vi "ADRextraction.vi"(8 "Path in":path) -> (10 "Error":string, 11 "Array":dbl[](array[numeric]), 12 "raw xML":string, 13 "duration":dbl[](array[numeric]), 14 "Start time":timestamp, 15 "Starttime":timestamp, 17 "currenttime":timestamp, 18 "End time":timestamp, 19 "Current time":timestamp, 21 "Price":dbl, 22 "error out 2":errorcluster, 23 "Numeric":dbl, 24 "error out":errorcluster, 25 "Endtime":timestamp, 27 "error out":errorcluster)   [LabVIEW 2020]
uses:
  <vilib>/xml/Close Reference(Node).vi
  <vilib>/xml/Close Reference(NdList).vi
  <vilib>/regexp/Match Regular Expression.xnode
  <vilib>/xml/NI_XML.lvlib
  <resource>/objmgr/DOMUserDefRef.rc
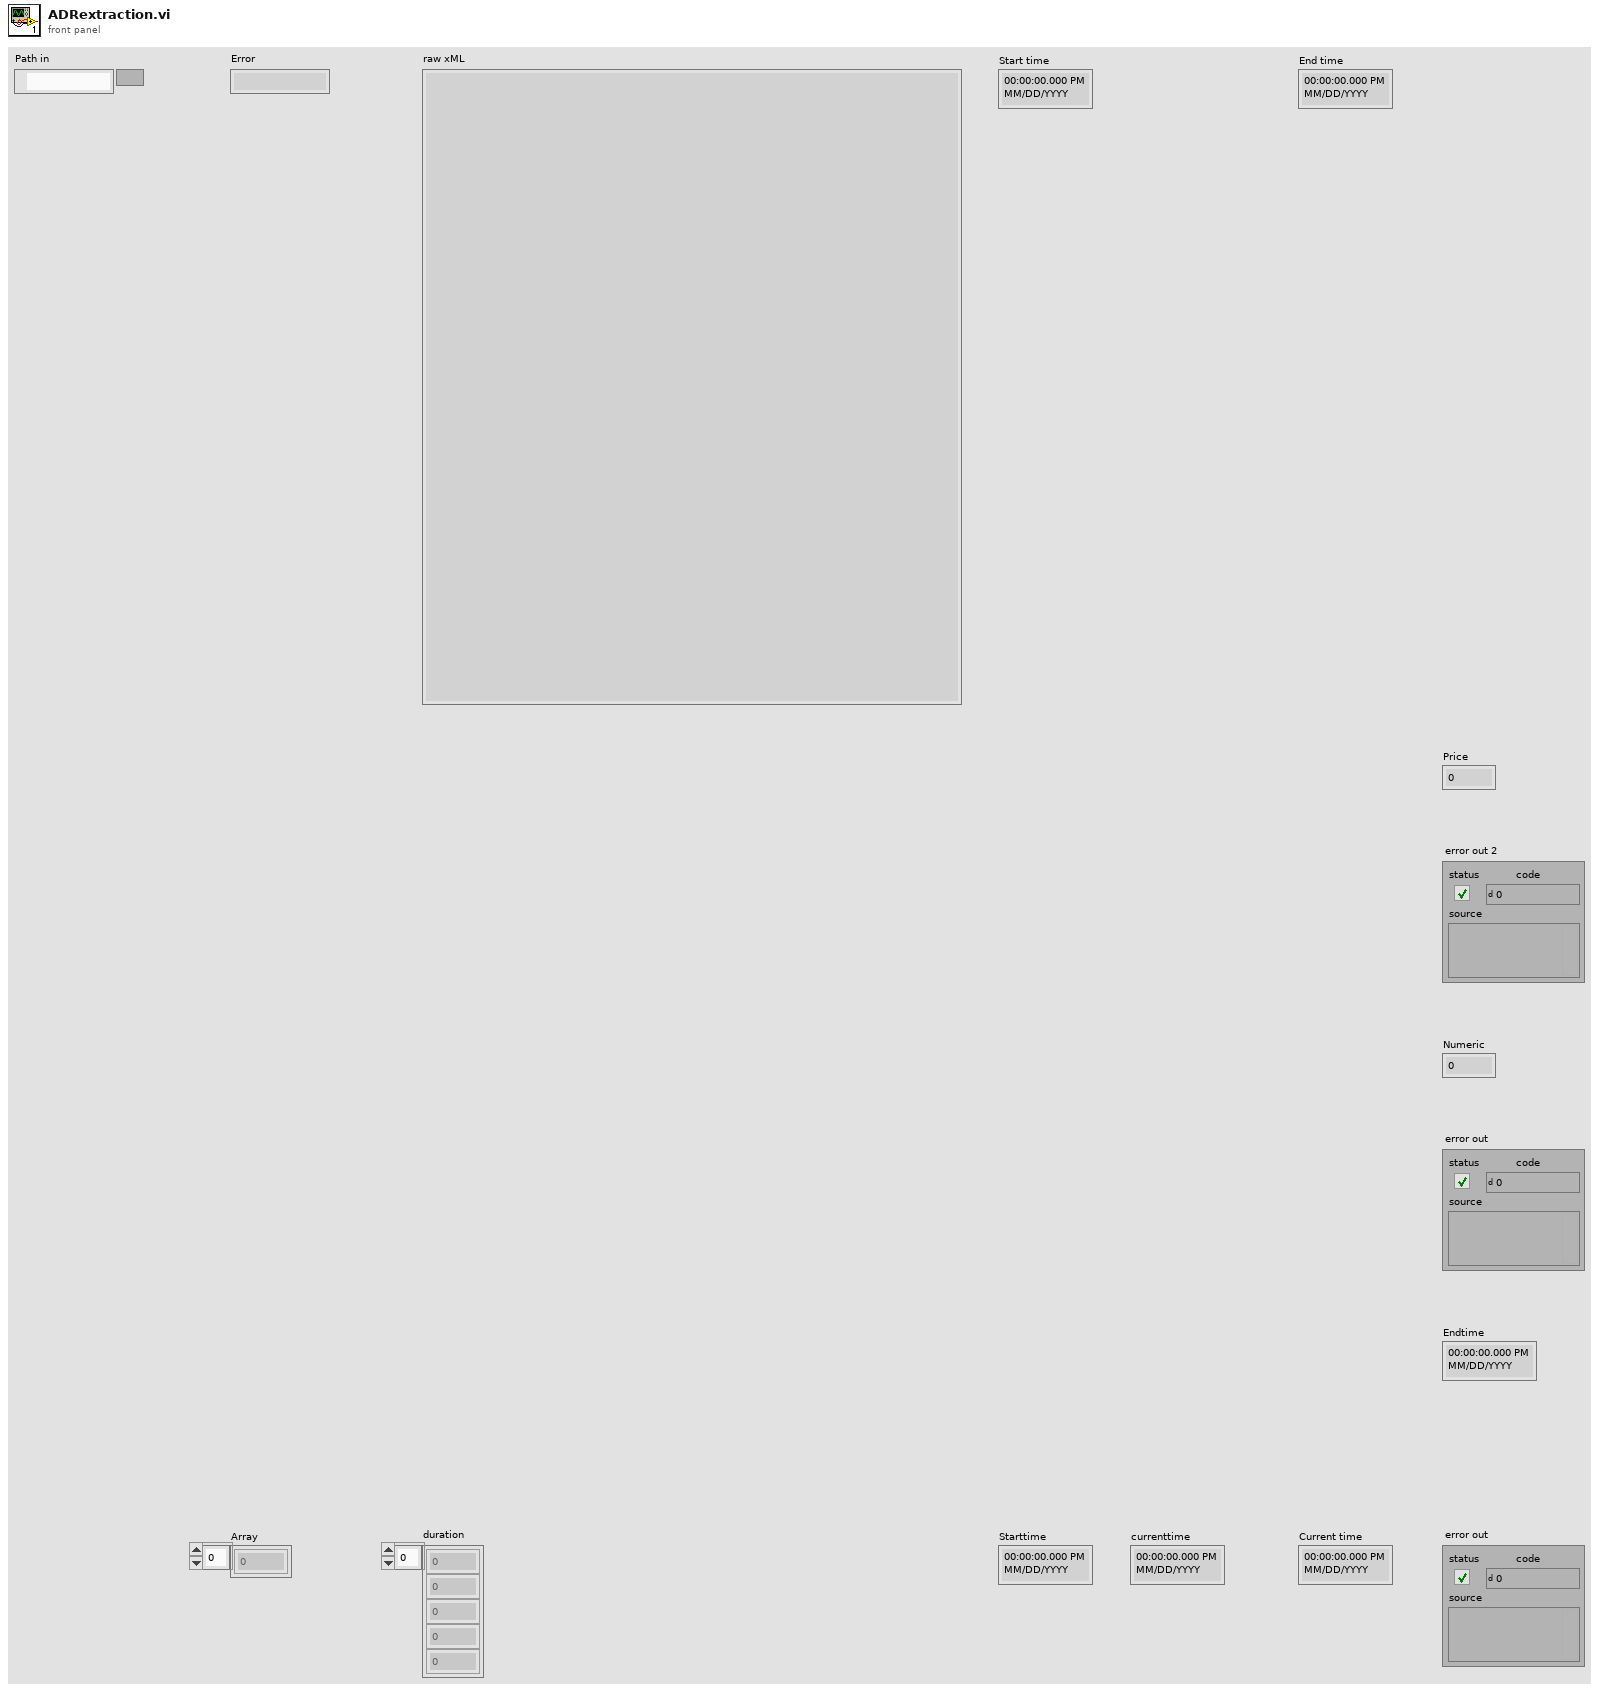
[diagram p1: front panel]
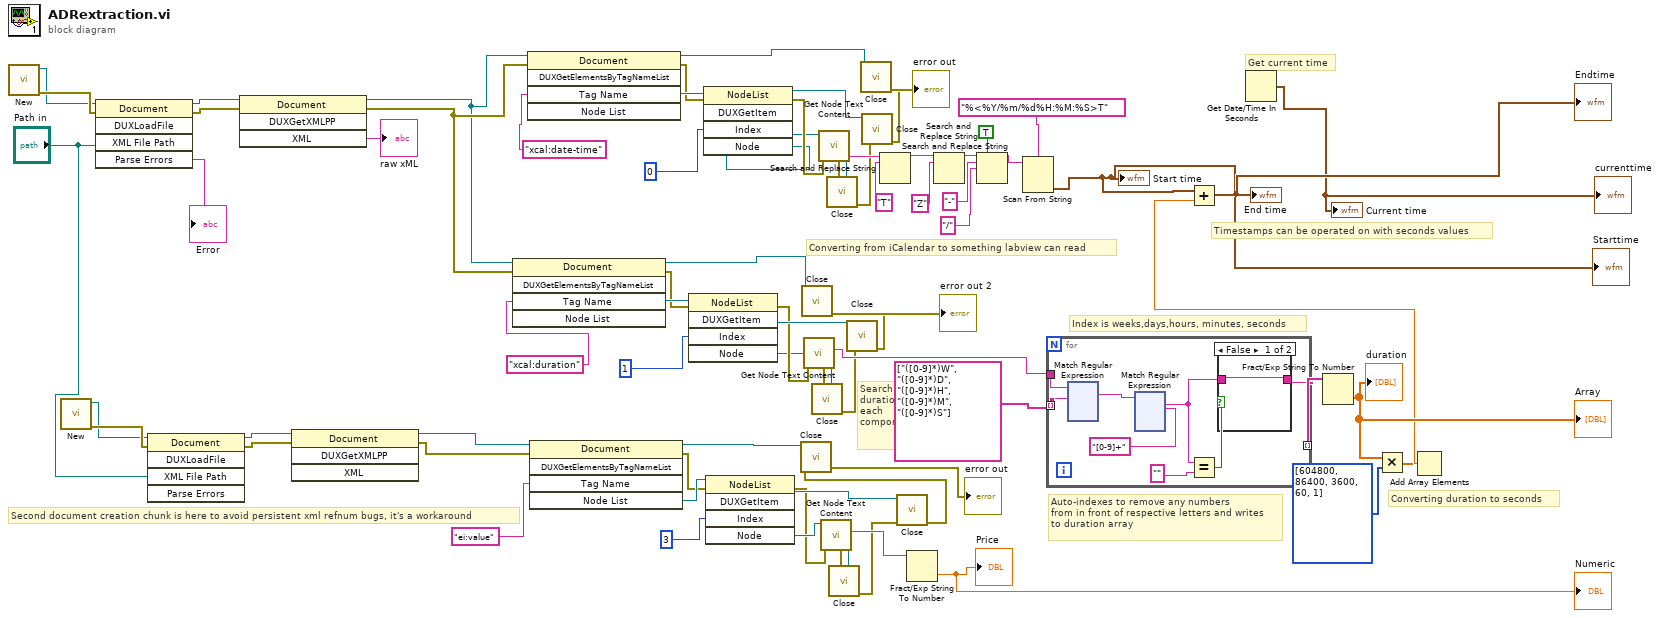
[diagram p0: block diagram]
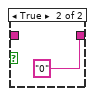
[diagram p2: hidden frame]
diagram:
  # "Timestamps can be operated on with seconds values"
  # "Auto-indexes to remove any numbers\nfrom in front of respective letters and writes\nto duration array"
  # "Converting from iCalendar to something labview can read"
  # "Second document creation chunk is here to avoid persistent xml refnum bugs, it's a workaround"
  # "Get current time"
  # "Converting duration to seconds"
  # "Search duration for each component"
  # "Index is weeks,days,hours, minutes, seconds"
  n1 = call <vilib>:"New.vi"() -> ("error out"=w2:errorcluster, "DOM document out"=w1:refnum<k20>)  [unwired: 8 in]
  n2 = call <vilib>:"New.vi"() -> ("error out"=w66:errorcluster, "DOM document out"=w65:refnum<k20>)  [unwired: 8 in]
  n3 = invoke class="Document" method="DUXLoadFile"(reference=w1, error in=w2, "XML File Path"="Path in") -> (reference out=w4:refnum<k20>, error out=w5:errorcluster, "Parse Errors"=→"Error":string)  [unwired: 2 in, 2 out]
  n4 = invoke class="Document" method="DUXLoadFile"(reference=w65, error in=w66, "XML File Path"="Path in") -> (reference out=w67:refnum<k20>, error out=w68:errorcluster)  [unwired: 2 in, 3 out]
  n5 = invoke class="Document" method="DUXGetXMLPP"(reference=w4, error in=w5) -> (reference out=w63:refnum<k20>, error out=w64:errorcluster, "XML"=→"raw xML":string)  [unwired: 2 in, 1 out]
  n6 = invoke class="Document" method="DUXGetXMLPP"(reference=w67, error in=w68) -> (reference out=w70:refnum<k20>, error out=w71:errorcluster)  [unwired: 2 in, 2 out]
  n7 = invoke class="Document" method="DUXGetElementsByTagNameList"(reference=w63, error in=w64, "Tag Name"="xcal:duration") -> (reference out=w21:refnum<k20>, error out=w26:errorcluster, "Node List"=w27:refnum<k20>)  [unwired: 2 in, 2 out]
  n8 = invoke class="Document" method="DUXGetElementsByTagNameList"(reference=w63, error in=w64, "Tag Name"="xcal:date-time") -> (reference out=w10:refnum<k20>, error out=w15:errorcluster, "Node List"=w16:refnum<k20>)  [unwired: 2 in, 2 out]
  n9 = invoke class="Document" method="DUXGetElementsByTagNameList"(reference=w70, error in=w71, "Tag Name"="ei:value") -> (reference out=w34:refnum<k20>, error out=w33:errorcluster, "Node List"=w60:refnum<k20>)  [unwired: 2 in, 2 out]
  n10 = invoke class="NodeList" method="DUXGetItem"(reference=w27, error in=w26, "Index"=1) -> (reference out=w28:refnum<k20>, error out=w25:errorcluster, "Node"=w24:refnum<k20>)  [unwired: 2 in, 2 out]
  n11 = invoke class="NodeList" method="DUXGetItem"(reference=w16, error in=w15, "Index"=0) -> (reference out=w17:refnum<k20>, error out=w14:errorcluster, "Node"=w13:refnum<k20>)  [unwired: 2 in, 2 out]
  n12 = invoke class="NodeList" method="DUXGetItem"(reference=w60, error in=w33, "Index"=3) -> (reference out=w44:refnum<k20>, error out=w43:errorcluster, "Node"=w62:refnum<k20>)  [unwired: 2 in, 2 out]
  n13 = call <vilib>:"Get Node Text Content.vi"("error in (no error)"=w25, "node in"=w24) -> ("error out"=w18:errorcluster, "node text"=w41:string, "node out"=w19:refnum<k20>)  [unwired: 7 in]
  n14 = call-poly <vilib>:"Close.vi"("error in (no error)"=w18, "node"=w19) -> ("error out"=w20:errorcluster)  [unwired: 7 in]
  n15 = call <vilib>:"Get Node Text Content.vi"("error in (no error)"=w14, "node in"=w13) -> ("error out"=w7:errorcluster, "node text"=w52:string, "node out"=w8:refnum<k20>)  [unwired: 7 in]
  n16 = call <vilib>:"Get Node Text Content.vi"("error in (no error)"=w43, "node in"=w62) -> ("error out"=w42:errorcluster, "node text"=w40:string, "node out"=w29:refnum<k20>)  [unwired: 7 in]
  n17 = call-poly <vilib>:"Close.vi"("error in (no error)"=w7, "node"=w8) -> ("error out"=w9:errorcluster)  [unwired: 7 in]
  n18 = call-poly <vilib>:"Close.vi"("error in (no error)"=w42, "node"=w29) -> ("error out"=w30:errorcluster)  [unwired: 7 in]
  n19 = call-poly <vilib>:"Close.vi"("error in (no error)"=w20, "node list"=w28) -> ("error out"=w22:errorcluster)  [unwired: 7 in]
  n20 = call-poly <vilib>:"Close.vi"("error in (no error)"=w22, "node"=w21) -> ("error out"=→"error out 2":errorcluster)  [unwired: 7 in]
  n21 = call-poly <vilib>:"Close.vi"("error in (no error)"=w9, "node list"=w17) -> ("error out"=w11:errorcluster)  [unwired: 7 in]
  n22 = call-poly <vilib>:"Close.vi"("error in (no error)"=w11, "node"=w10) -> ("error out"=→"error out":errorcluster)  [unwired: 7 in]
  n23 = Search and Replace String(input string=w52, search string="T") -> (result string=w45:string)  [unwired: 6 in, 3 out]
  n24 = call-poly <vilib>:"Close.vi"("error in (no error)"=w30, "node list"=w44) -> ("error out"=w31:errorcluster)  [unwired: 7 in]
  n25 = call-poly <vilib>:"Close.vi"("error in (no error)"=w31, "node"=w34) -> ("error out"=→"error out":errorcluster)  [unwired: 7 in]
  n26 = Fract/Exp String To Number(string=w40) -> (number=→"Price" →"Numeric":dbl)  [unwired: 3 in, 1 out]
  n27 = Search and Replace String(input string=w45, search string="Z") -> (result string=w47:string)  [unwired: 6 in, 3 out]
  n28 = Search and Replace String(replace all?=TRUE, input string=w47, search string="-", replace string="/") -> (result string=w59:string)  [unwired: 4 in, 3 out]
  n29 = Scan From String(format string="%<%Y/%m/%d%H:%M:%S>T", input string=w59) -> (output 1=w73:timestamp)  [unwired: 3 in, 3 out]
  "Start time" <- w73
  "Starttime" <- w73
  n30 = for {
    tunnel: string[] ["([0-9]*)W", "([0-9]*)D", "([0-9]*)H", "([0-9]*)M", "([0-9]*)S"] -> [w84] mode=indexing
    tunnel: w41 -> [w83]
    tunnel: [w77] -> w54 mode=indexing
    n31 = xnode "Match Regular Expression"("input string"=w83, "regular expression"=w84) -> ("whole match"=w82:string)  [unwired: 4 in, 4 out]
    n32 = xnode "Match Regular Expression"("input string"=w82, "regular expression"="[0-9]+") -> ("whole match"=w78:string)  [unwired: 4 in, 4 out]
    n33 = Equal?(x=w78, y="") -> (x = y?=w79:bool)
    n34 = case shown="False" w79 {
      tunnel: [w85 "0"] -> w77
      tunnel: w78 -> [w85 _]
      frame False {
      }
      frame True {
      }
    }
  }
  n35 = Get Date/Time In Seconds() -> (seconds since 1Jan1904=→"Current time" →"currenttime":timestamp)
  n36 = Fract/Exp String To Number(string=w54) -> (number=w75:dbl[])  [unwired: 3 in, 1 out]
  "duration" <- w75
  "Array" <- w75
  n37 = Multiply(x=w75, y=i32[] [604800, 86400, 3600, 60, 1]) -> (x*y=w57:dbl[])
  n38 = Add Array Elements(numeric array=w57) -> (sum=w58:dbl)
  n39 = Add(x=w73, y=w58) -> (x+y=→"End time" →"Endtime":timestamp)
